vi "Temperature Warnings.vi"() -> ()   [LabVIEW 2020]
panel:
  out "Error Out":errorcluster
  in  "Error In":errorcluster
  out "Warning?":bool
  out "Warning Text":string
  in  "Min Temperature":dbl
  in  "Max Temperature":dbl
  in  "Current Temperature":dbl
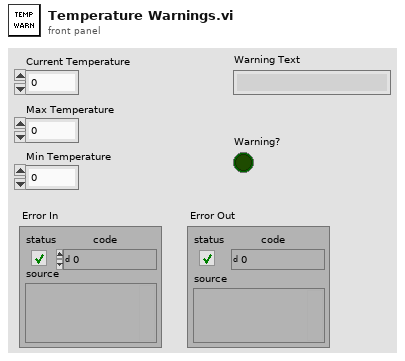
[diagram p1: front panel]
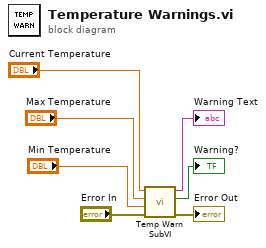
[diagram p0: block diagram]
diagram:
  n1 = call "Temp Warn SubVI.vi"("error in (no error)"="Error In", "Min Temperature"="Min Temperature", "Max Temperature"="Max Temperature", "Current Temperature"="Current Temperature") -> ("error out"=→"Error Out":errorcluster, "Boolean"=→"Warning?":bool, "f"=→"Warning Text":string)  [unwired: 5 in]
